vi "Sub_LEMP2.vi"(1 "Pin-Location":i32, 2 "Beam Model":T1) -> (0 "eigenvalues updated":dbl[](array[numeric]))   [LabVIEW 2019]
uses:
  LabVIEW_FEA_simulation 2022/Main_code/secular_solver/bin/Debug/secular_solver.dll
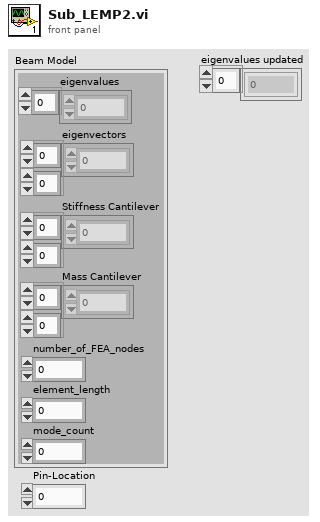
[diagram p1: front panel]
types:
  T1 = cluster{"eigenvalues":dbl[], "element_length ":dbl, "number_of_FEA_nodes":i32, "Stiffness Cantilever":dbl[][], "Mass Cantilever":dbl[][], "eigenvectors":dbl[][], "mode_count":i32}
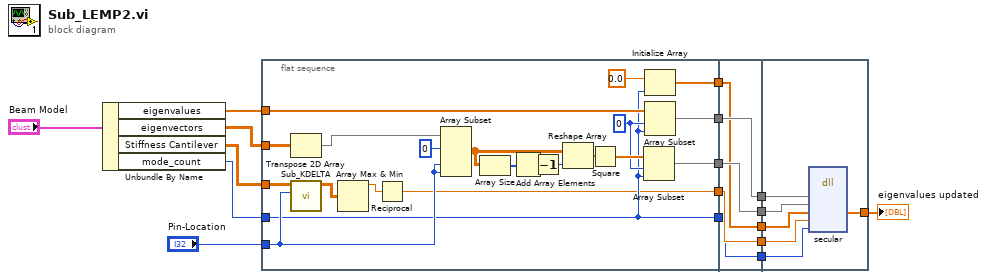
[diagram p0: block diagram]
diagram:
  n1 = Unbundle By Name("Beam Model") -> ("eigenvalues"=w4:dbl[], "eigenvectors"=w3:dbl[][], "Stiffness Cantilever"=w2:dbl[][], "mode_count"=w1:i32)
  n2 = flat-sequence {
    tunnel: w3 -> [w38]
    tunnel: w2 -> [w37]
    tunnel: "Pin-Location" -> [w32]
    tunnel: w4 -> [w25]
    tunnel: w1 -> [w19]
    tunnel: [w22] -> w16
    tunnel: [w21] -> w15
    tunnel: [w20] -> w14
    tunnel: [w19] -> w13
    tunnel: [w18] -> w12
    tunnel: w16 -> [w41]
    tunnel: w15 -> [w43]
    tunnel: w14 -> [w42]
    tunnel: w13 -> [w39]
    tunnel: w12 -> [w40]
    tunnel: [w43] -> w11
    tunnel: [w42] -> w10
    tunnel: [w41] -> w9
    tunnel: [w40] -> w8
    tunnel: [w39] -> w7
    tunnel: w11 -> [w49]
    tunnel: w10 -> [w48]
    tunnel: w9 -> [w47]
    tunnel: w8 -> [w46]
    tunnel: w7 -> [w45]
    tunnel: [w44] -> w6
    frame #0 {
      w23 = 0 ("index")
      n3 = Transpose 2D Array(2D array=w38) -> (transposed array=w34:dbl[][])
      n4 = call "Sub_KDELTA.vi"("Pin-Location"=w32, "Pre-Pin Matrix"=w37) -> ("Pin-Delta Matrix"=w36:dbl[][])  [unwired: 8 in]
      n5 = Array Max & Min(array=w36) -> (max value=w35:dbl)  [unwired: 3 out]
      n6 = Reciprocal(x=w35) -> (1/x=w18:dbl)
      n7 = Array Subset(array=w34, index (row)=0 ("row 1"), index (col)=w32, length (col)=w32) -> (w28:dbl[][])  [unwired: 1 in]
      n8 = Array Size(array=w28) -> (size(s)=w31:i32[])
      n9 = Add Array Elements(numeric array=w31) -> (sum=w30:i32)
      n10 = Decrement(x=w30) -> (x-1=w29:i32)
      n11 = Reshape Array(w28, w29) -> (w27:dbl[])
      n12 = Square(x=w27) -> (x^2=w26:dbl[])
      n13 = Array Subset(array=w26, index=w23, length=w19) -> (w20:dbl[])
      n14 = Initialize Array(0.0 ("element"), w19) -> (w22:dbl[])
      n15 = Array Subset(array=w25, index=w23, length=w19) -> (w21:dbl[])
    }
    frame #1 {
    }
    frame #2 {
      n16 = dll-call lib="C:/Users/PXIe-8880/Documents/AFRL_summer_2022/LabVIEW_FEA_simulation 2022/Main_code/secular_solver/bin/Debug/secular_solver.dll" fn="secular"("d"=w49, "v"=w48, "sol"=w47, "p"=w46, "mode"=w45) -> ("sol"=w44:dbl[])  [unwired: 8 in, 2 out]
    }
  }
  "eigenvalues updated" <- w6
